vi "Range of Left Side.vi"(10 "offsetAngle V":dbl, 11 "offsetAngle H":dbl) -> (3 "Boolean":bool)   [LabVIEW 2023]
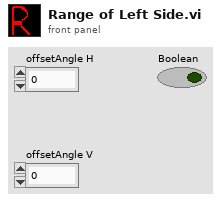
[diagram p1: front panel]
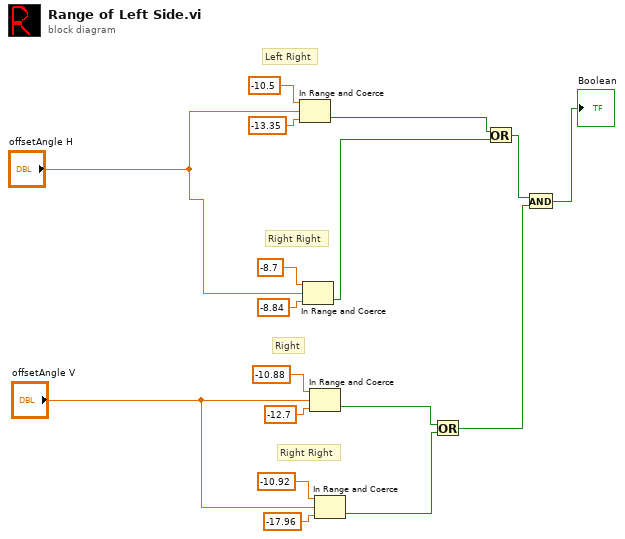
[diagram p0: block diagram]
diagram:
  # "Right Right"
  # "Right"
  # "Right Right"
  # "Left Right"
  n1 = In Range and Coerce(upper limit=-10.5, x="offsetAngle H", lower limit=-13.35) -> (In Range?=w10:bool)  [unwired: 1 out]
  n2 = In Range and Coerce(upper limit=-8.7, x="offsetAngle H", lower limit=-8.84) -> (In Range?=w9:bool)  [unwired: 1 out]
  n3 = In Range and Coerce(upper limit=-10.88, x="offsetAngle V", lower limit=-12.7) -> (In Range?=w3:bool)  [unwired: 1 out]
  n4 = In Range and Coerce(upper limit=-10.92, x="offsetAngle V", lower limit=-17.96) -> (In Range?=w2:bool)  [unwired: 1 out]
  n5 = Or(x=w3, y=w2) -> (x .or. y?=w1:bool)
  n6 = Or(x=w10, y=w9) -> (x .or. y?=w7:bool)
  n7 = And(x=w7, y=w1) -> (x .and. y?=→"Boolean":bool)
